vi "BME_DG_Set_G05_Chnl.vi"(8 "error in (no error)":errorcluster, 9 "ChnParameter":T1={" Delay (µs)"=0.0, "TriggerModulo"=1, "On? (false)"=FALSE, "PositiveVoltage?(true)"=FALSE, "50OhmTerminated? "=FALSE, "25OhmOutput?"=FALSE} {"TriggerModulo" min=1 max=1000000; "Delay (µs)" min=0.0 max=100000000.0 format="%.5f"}, 10 "Channel":u32=1, 11 "DG_Number":i32) -> (0 "error out":errorcluster, 3 "return code":i32)   [LabVIEW 2009, in "POLARIS BME DG.lvlib"]
uses:
  POLARIS BME DG.lvlib
  ChnlWithModulo.ctl
  BME DLL/DelayGenerator.dll
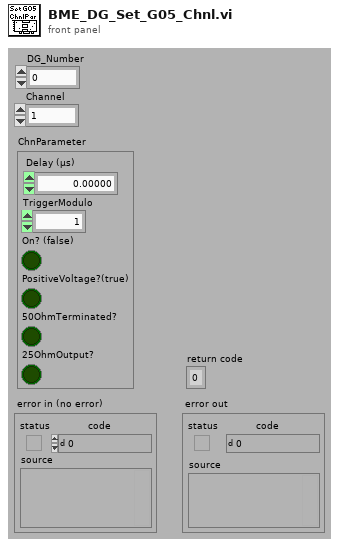
[diagram p1: front panel]
types:
  T1 = typedef "POLARIS BME DG.lvlib/ChnlWithModulo.ctl" = cluster{" Delay (µs)":dbl, "TriggerModulo":u32, "On? (false)":bool, "PositiveVoltage?(true)":bool, "50OhmTerminated? ":bool, "25OhmOutput?":bool}
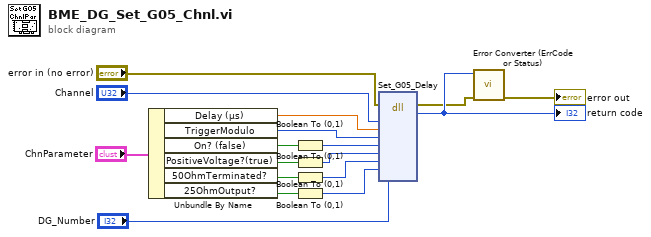
[diagram p0: block diagram]
diagram:
  n1 = Unbundle By Name("ChnParameter") -> ("Delay (µs)"=w12:dbl, "TriggerModulo"=w4:u32, "On? (false)"=w11:bool, "PositiveVoltage?(true)"=w10:bool, "50OhmTerminated?"=w9:bool, "25OhmOutput?"=w8:bool)
  n2 = Boolean To (0,1)(Boolean=w11) -> (0, 1=w16:i16)
  n3 = Boolean To (0,1)(Boolean=w10) -> (0, 1=w15:i16)
  n4 = Boolean To (0,1)(Boolean=w9) -> (0, 1=w14:i16)
  n5 = Boolean To (0,1)(Boolean=w8) -> (0, 1=w13:i16)
  n6 = dll-call lib="C:/CS Framework/LVSCC/LV2009/GPL/Projects/cs-framework/CSClass/CSPOLARIS/POLARIS BME DG/BME DLL/DelayGenerator.dll" fn="Set_G05_Delay"(error in="error in (no error)", "Channel"="Channel", "FireFirst"=w12, "Modulo"=w4, "Active"=w16, "Positive"=w15, "Terminate"=w14, "HighDrive"=w13, "DG_Number"="DG_Number") -> (error out=w2:errorcluster, "Error"=w3:i32)  [unwired: 10 in, 1 out]
  "return code" <- w3
  n7 = call "Error Converter (ErrCode or Status).vi"("error in (no error)"=w2, "error code"=w3) -> ("error out"=→"error out":errorcluster)  [unwired: 9 in]
